vi "Limited Integrator.vi"   [LabVIEW 2017, in "NI_AdvCtrl_continuous linear.lvlib"]
doc: "LabVIEW no longer supports this VI. You can obtain similar functionality by installing the LabVIEW Simulation Module.\n\nIntegrates a continuous input signal where limits are given. The integration process is based on Euler method. dt must be positive. The result of the integration process is in between of lower bound and upper bound."
uses:
  <vilib>/addons/control/advanced/NI_AdvCtrl_continuous linear.lvlib
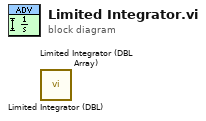
[diagram p0: block diagram]
diagram:
  n1 = call <vilib>:"Limited Integrator (DBL).vi"() -> ()  [unwired: 10 in, 1 out]
  n2 = call <vilib>:"Limited Integrator (DBL Array).vi"() -> ()  [unwired: 10 in, 1 out]
